vi "Copy State.vi"(6 "Already Exist Action:\nReplace(T) / Skip(F)":bool, 7 "SourceCSM":refnum<class "CSM-Helper.lvclass">=refnum, 8 "error in (no error)":errorcluster, 9 "New(Empty to Use same Name)":string, 10 "Case":string="UI: Cursor Set", 11 "CSM-Helper.lvclass":refnum<class "CSM-Helper.lvclass">=refnum) -> (0 "error out":errorcluster, 3 "CSM-Helper out 2":refnum<class "CSM-Helper.lvclass">)   [LabVIEW 2017, in "CSM-Helper.lvclass"]
doc: "### Copy State.vi\n\n-- <b>Controls</b> --\n- <b>Already Exist Action:\nReplace(T) / Skip(F)</b>:\n- <b>SourceCSM</b>:\n- <b>New(Empty to Use same Name)</b>:\n- <b>Case</b>:\n- <b>CSM-Helper.lvclass</b>:\n\n-- <b>Indicators</b> --\n- <b>CSM-Helper out 2</b>:"
uses:
  CSM-Helper.lvclass
  <vilib>/Utility/miscctls.llb/LVPositionTypeDef.ctl
  CSM-Helper.lvclass/CSM-Helper.ctl
  Properties/Read Case Structure Ref.vi
  Properties/Read States.vi
  Remove State Frame.vi
  Get CaseFrame Reference By CaseName.vi
  Properties/Read Block Diagram Ref.vi
  Connect Internal Data Wire If not Connected.vi
  Connect StateQ Wire If not Connected.vi
  Connect Error Wire If not Connected.vi
  Connect Paired Tunnels.vi
  Utility/_Support/Diagram.llb/csmHelper-Diagram.lvlib
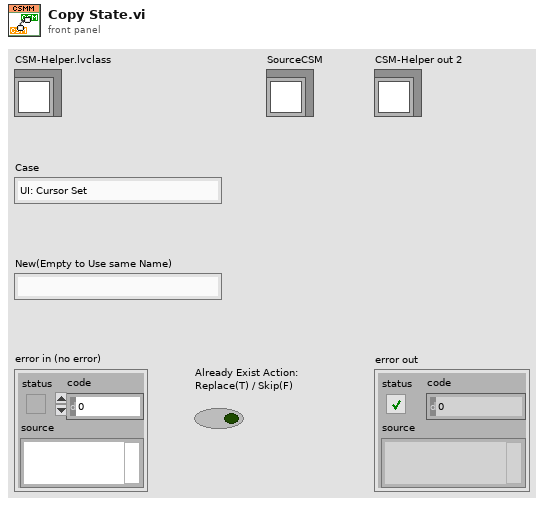
[diagram p1: front panel]
types:
  T1 = typedef "LVPositionTypeDef.ctl" = cluster{"Left":i32, "Top":i32}
  T2 = typedef "LVBoundsTypeDef.ctl" = cluster{"Width":u32, "Height":u32}
  T3 = typedef "csmHelper-Diagram.lvlib/Def-Conncted Information.ctl" = cluster{"Node Index":i32, "Tunnel Relative Pos":T1, "Term Index":i32, "ObjClassName":string, "OwnerClassName":string}
  T4 = cluster{"Registration":refnum<vi>, "InternalData":refnum<vi>, "CSM Name":refnum<vi>, "Last Resp":refnum<vi>, "Remaining State":refnum<vi>, "Arguments":refnum<vi>, "Response Source":refnum<vi>, "Source CSM":refnum<vi>, "Selector":refnum<vi>, "Error":refnum<vi>}
  T5 = cluster{"Registration":refnum<vi>, "InternalData":refnum<vi>, "Resp":refnum<vi>, "Remaining State":refnum<vi>, "Error":refnum<vi>}
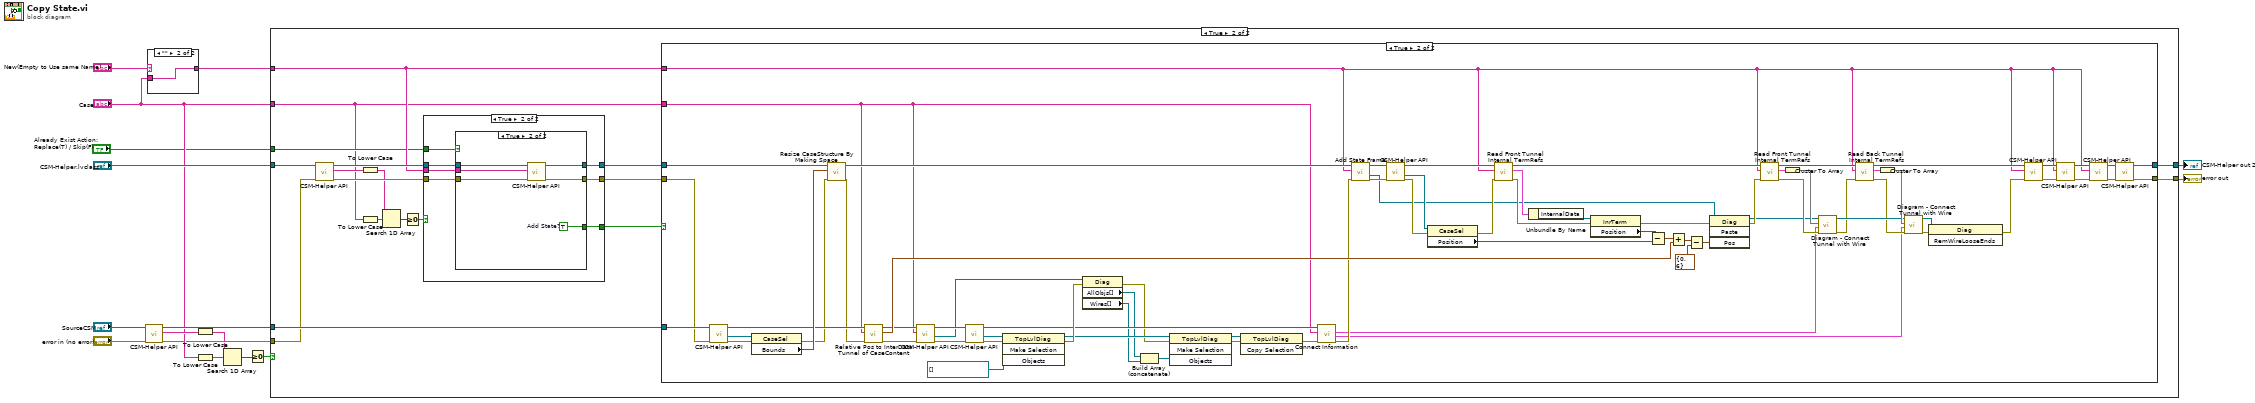
[diagram p0: block diagram]
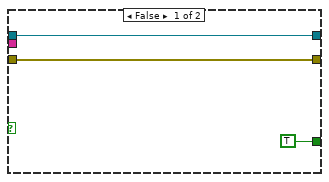
[diagram p4: hidden frame]
diagram:
  n1 = call-poly "CSM-Helper API.vi"("error in (no error)"="error in (no error)", "CSM-Helper in"="SourceCSM") -> ("error out"=w5:errorcluster, "Value"=w8:string[], "CSM-Helper out"=w10:refnum<class "CSM-Helper.lvclass">)  [unwired: 7 in]
  n2 = case shown="\"\"" "New(Empty to Use same Name)" {
    selector: "New(Empty to Use same Name)" -> [w17 _]
    tunnel: [w17 w18] -> w13
    tunnel: "Case" -> [_ w18]
    frame "False", Default {
    }
    frame "" {
    }
  }
  n3 = To Lower Case(string=w8) -> (all lower case string=w2:string[])
  n4 = To Lower Case(string="Case") -> (all lower case string=w1:string)
  n5 = Search 1D Array(1D array=w2, element=w1) -> (index of element=w6:i32)  [unwired: 1 in]
  n6 = Greater Or Equal To 0?(x=w6) -> (x >= 0?=w4:bool)
  n7 = case shown="True" w4 {
    tunnel: "CSM-Helper.lvclass" -> [w19 w38]
    tunnel: w13 -> [_ w28]
    tunnel: [w19 w37] -> w12
    tunnel: [w20 w36] -> w11
    tunnel: w10 -> [_ w35]
    tunnel: "Case" -> [_ w23]
    tunnel: w5 -> [w20 w34]
    tunnel: "Already Exist Action:\nReplace(T) / Skip(F)" -> [_ w25]
    frame False {
    }
    frame True {
      n8 = call-poly "CSM-Helper API.vi"("error in (no error)"=w34, "CSM-Helper in"=w38) -> ("error out"=w27:errorcluster, "Value"=w32:string[], "CSM-Helper out"=w31:refnum<class "CSM-Helper.lvclass">)  [unwired: 7 in]
      n9 = To Lower Case(string=w32) -> (all lower case string=w22:string[])
      n10 = To Lower Case(string=w23) -> (all lower case string=w21:string)
      n11 = Search 1D Array(1D array=w22, element=w21) -> (index of element=w33:i32)  [unwired: 1 in]
      n12 = Greater Or Equal To 0?(x=w33) -> (x >= 0?=w30:bool)
      n13 = case shown="True" w30 {
        tunnel: w31 -> [w117 w125]
        tunnel: [w117 w124] -> w29
        tunnel: w28 -> [_ w123]
        tunnel: w27 -> [w118 w122]
        tunnel: [w118 w121] -> w26
        tunnel: w25 -> [_ w120]
        tunnel: [TRUE ("Add State?") w119] -> w24
        frame False {
        }
        frame True {
          n14 = case shown="True" w120 {
            tunnel: w125 -> [w127 w133]
            tunnel: [w127 w132] -> w124
            tunnel: w123 -> [_ w131]
            tunnel: w122 -> [w126 w130]
            tunnel: [w126 w129] -> w121
            tunnel: [_ w128] -> w119
            frame False {
            }
            frame True {
              w128 = TRUE  # Add State?
              n15 = call-poly "CSM-Helper API.vi"("error in (no error)"=w130, "element"=w131, "CSM-Helper in"=w133) -> ("error out"=w129:errorcluster, "CSM-Helper out"=w132:refnum<class "CSM-Helper.lvclass">)  [unwired: 7 in]
            }
          }
        }
      }
      n16 = case shown="True" w24 {
        tunnel: [w39 w47] -> w37
        tunnel: [w40 w46] -> w36
        tunnel: w35 -> [_ w45]
        tunnel: w23 -> [_ w44]
        tunnel: w29 -> [w39 w43]
        tunnel: w28 -> [_ w42]
        tunnel: w26 -> [w40 w41]
        frame False {
        }
        frame True {
          n17 = call-poly "CSM-Helper API.vi"("error in (no error)"=w41, "CSM-Helper in"=w45) -> ("error out"=w70:errorcluster, "Case Structure"=w64:refnum<vi>, "CSM-Helper out"=w69:refnum<class "CSM-Helper.lvclass">)  [unwired: 7 in]
          n18 = property on="Property Node" class="CaseSel"(reference=w64, error in=w70) -> (error out=w68:errorcluster, "Bounds"=w72:T2)  [unwired: 1 out]
          n19 = call "Resize CaseStructure By Making Space.vi"("error in (no error)"=w68, "Bounds"=w72, "CSM-Helper in"=w43) -> ("error out"=w67:errorcluster, "CSM-Helper out"=w71:refnum<class "CSM-Helper.lvclass">)  [unwired: 5 in, 2 out]
          n20 = call "Relative Pos to InterData Tunnel of CaseContent.vi"("error in (no error)"=w67, "element"=w44, "CSM-Helper in"=w69) -> ("error out"=w79:errorcluster, "Position"=w101:T1, "CSM-Helper out"=w76:refnum<class "CSM-Helper.lvclass">)  [unwired: 6 in]
          n21 = call-poly "CSM-Helper API.vi"("error in (no error)"=w79, "CASE"=w44, "CSM-Helper in"=w76) -> ("error out"=w78:errorcluster, "Frame Refs"=w65:refnum<vi>, "CSM-Helper out"=w77:refnum<class "CSM-Helper.lvclass">)  [unwired: 6 in]
          n22 = call-poly "CSM-Helper API.vi"("error in (no error)"=w78, "CSM-Helper in"=w77) -> ("error out"=w74:errorcluster, "Diagram"=w66:refnum<vi>, "CSM-Helper out"=w61:refnum<class "CSM-Helper.lvclass">)  [unwired: 7 in]
          n23 = invoke on="Invoke Node" class="TopLvlDiag" method="Make Selection"(reference=w66, error in=w74, "Objects"=refnum<vi>[] []) -> (reference out=w56:refnum<vi>, error out=w75:errorcluster)  [unwired: 1 in, 2 out]
          n24 = property class="Diag"(reference=w65, error in=w75) -> (error out=w54:errorcluster, "AllObjs[]"=w52:refnum<vi>[], "Wires[]"=w50:refnum<vi>[])  [unwired: 1 out]
          n25 = Build Array (concatenate)(w52, w50) -> (w51:refnum<vi>[])
          n26 = invoke on="Invoke Node" class="TopLvlDiag" method="Make Selection"(reference=w56, error in=w54, "Objects"=w51) -> (reference out=w55:refnum<vi>, error out=w53:errorcluster)  [unwired: 1 in, 2 out]
          n27 = invoke on="Invoke Node" class="TopLvlDiag" method="Copy Selection"(reference=w55, error in=w53) -> (error out=w81:errorcluster)  [unwired: 1 in, 2 out]
          n28 = call "Connect Information.vi"("error in (no error)"=w81, "Case"=w44, "CSM-Helper in"=w61) -> ("error out"=w80:errorcluster, "Backend Connected Info"=w59:T3[], "FrontEnd Connected Info"=w60:T3[])  [unwired: 5 in, 1 out]
          n29 = call "Add State Frame.vi"("error in (no error)"=w80, "element"=w42, "CSM-Helper in"=w71) -> ("error out"=w108:errorcluster, "Add Frame"=w62:refnum<vi>, "CSM-Helper out"=w114:refnum<class "CSM-Helper.lvclass">)  [unwired: 6 in]
          n30 = call-poly "CSM-Helper API.vi"("error in (no error)"=w108, "CSM-Helper in"=w114) -> ("error out"=w83:errorcluster, "Case Structure"=w63:refnum<vi>, "CSM-Helper out"=w109:refnum<class "CSM-Helper.lvclass">)  [unwired: 7 in]
          n31 = property on="Property Node" class="CaseSel"(reference=w63, error in=w83) -> (error out=w82:errorcluster, "Position"=w104:T1)  [unwired: 1 out]
          n32 = call "Read Front Tunnel Internal TermRefs.vi"("error in (no error)"=w82, "case"=w42, "CSM-Helper in"=w109) -> ("error out"=w112:errorcluster, "Front Tunnels"=w111:T4, "CSM-Helper out"=w110:refnum<class "CSM-Helper.lvclass">)  [unwired: 6 in]
          n33 = Unbundle By Name(w111) -> ("InternalData"=w115:refnum<vi>)
          n34 = property on="Property Node" class="InrTerm"(reference=w115, error in=w112) -> (error out=w113:errorcluster, "Position"=w105:T1)  [unwired: 1 out]
          n35 = Subtract(x=w105, y=w104) -> (x-y=w107:T1)
          n36 = Add(x=w107, y=w101) -> (x+y=w106:T1)
          n37 = Subtract(x=w106, y=T1 {"Left"=0, "Top"=6}) -> (x-y=w103:T1)
          n38 = invoke on="Invoke Node" class="Diag" method="Paste"(reference=w62, error in=w113, "Pos"=w103) -> (reference out=w57:refnum<vi>, error out=w58:errorcluster)  [unwired: 1 in, 2 out]
          n39 = call "Read Front Tunnel Internal TermRefs.vi"("error in (no error)"=w58, "case"=w42, "CSM-Helper in"=w110) -> ("error out"=w99:errorcluster, "Front Tunnels"=w98:T4, "CSM-Helper out"=w96:refnum<class "CSM-Helper.lvclass">)  [unwired: 6 in]
          n40 = Cluster To Array(cluster=w98) -> (array=w100:refnum<vi>[])
          n41 = call "Diagram - Connect Tunnel with Wire.vi"("error in (no error)"=w99, "FrontEnd Connected Info"=w60, "Front Tunnels"=w100, "Diagram in"=w57) -> ("error out"=w89:errorcluster, "Diagram out"=w91:refnum<vi>)  [unwired: 5 in, 1 out]
          n42 = call "Read Back Tunnel Internal TermRefs.vi"("error in (no error)"=w89, "element"=w42, "CSM-Helper in"=w96) -> ("error out"=w88:errorcluster, "Back Tunnels"=w97:T5, "CSM-Helper out"=w95:refnum<class "CSM-Helper.lvclass">)  [unwired: 6 in]
          n43 = Cluster To Array(cluster=w97) -> (array=w92:refnum<vi>[])
          n44 = call "Diagram - Connect Tunnel with Wire.vi"("error in (no error)"=w88, "FrontEnd Connected Info"=w59, "Front Tunnels"=w92, "Diagram in"=w91) -> ("error out"=w90:errorcluster, "Diagram out"=w84:refnum<vi>)  [unwired: 5 in, 1 out]
          n45 = invoke on="Invoke Node" class="Diag" method="RemWireLooseEnds"(reference=w84, error in=w90) -> (error out=w85:errorcluster)  [unwired: 1 in, 2 out]
          n46 = call-poly "CSM-Helper API.vi"("error in (no error)"=w85, "case"=w42, "CSM-Helper in"=w95) -> ("error out"=w94:errorcluster, "CSM-Helper out"=w93:refnum<class "CSM-Helper.lvclass">)  [unwired: 7 in]
          n47 = call-poly "CSM-Helper API.vi"("error in (no error)"=w94, "case"=w42, "CSM-Helper in"=w93) -> ("error out"=w86:errorcluster, "CSM-Helper out"=w87:refnum<class "CSM-Helper.lvclass">)  [unwired: 7 in]
          n48 = call-poly "CSM-Helper API.vi"("error in (no error)"=w86, "case"=w42, "CSM-Helper in"=w87) -> ("error out"=w49:errorcluster, "CSM-Helper out"=w48:refnum<class "CSM-Helper.lvclass">)  [unwired: 7 in]
          n49 = call-poly "CSM-Helper API.vi"("error in (no error)"=w49, "CSM-Helper in"=w48) -> ("error out"=w46:errorcluster, "CSM-Helper out"=w47:refnum<class "CSM-Helper.lvclass">)  [unwired: 8 in]
        }
      }
    }
  }
  "CSM-Helper out 2" <- w12
  "error out" <- w11
